vi "bigEncoder3.vi"(4 "Positive Direction":bool, 5 "ForceReset":bool, 7 "Allow C Reset?":bool=TRUE, 8 "Reset Array":bool[](array[boolean])=[FALSE, FALSE, FALSE], 11 "Encoder Array":bool[](array[boolean])=[FALSE, FALSE, FALSE]) -> (0 "Reseting":bool, 1 "JumpBy2Bit":bool, 2 "JumpBy2Error":i16, 3 "Position":i32)   [LabVIEW 2016, in "KevLib01.lvlib"]
uses:
  KevLib01.lvlib
panel:
  # "The Main Difference is I added Allowable C Reset"
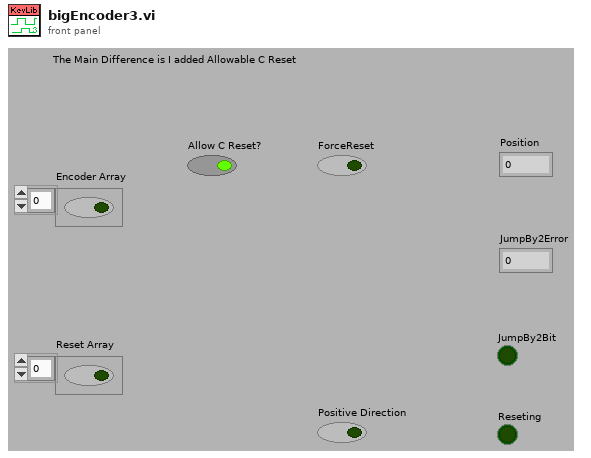
[diagram p1: front panel]
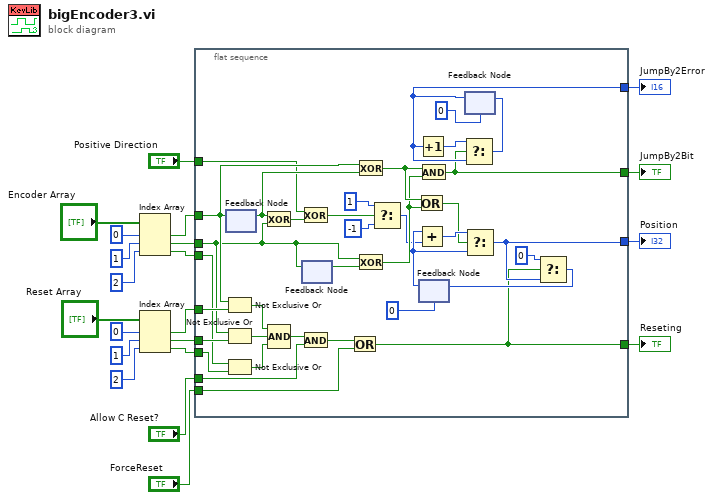
[diagram p0: block diagram]
diagram:
  n1 = Index Array(array="Encoder Array", index #1=0 ("index"), index #2=1 ("index"), index #3=2 ("index")) -> (element #1=w9:bool, element #2=w8:bool, element #3=w7:bool)
  n2 = Index Array(array="Reset Array", index #1=0 ("index"), index #2=1 ("index"), index #3=2 ("index")) -> (element #1=w6:bool, element #2=w5:bool, element #3=w4:bool)
  n3 = flat-sequence {
    tunnel: w9 -> [w37]
    tunnel: w8 -> [w35]
    tunnel: [w42] -> w21
    tunnel: [w45] -> w20
    tunnel: "ForceReset" -> [w39]
    tunnel: w6 -> [w38]
    tunnel: w5 -> [w36]
    tunnel: w4 -> [w34]
    tunnel: w7 -> [w33]
    tunnel: "Positive Direction" -> [w27]
    tunnel: [w26] -> w3
    tunnel: [w25] -> w2
    tunnel: "Allow C Reset?" -> [w23]
    frame #0 {
      n4 = Not Exclusive Or(1:w38, 2:w37) -> (0:w32:bool)
      n5 = Not Exclusive Or(1:w36, 2:w35) -> (0:w31:bool)
      n6 = Not Exclusive Or(1:w34, 2:w33) -> (0:w30:bool)
      n7 = feedback-in #1(w37) -> ()
      n8 = feedback #1() -> (w56:bool)  [unwired: 1 out]
      n9 = Exclusive Or(1:w35, 2:w56) -> (0:w29:bool)
      n10 = Compound Arithmetic op=AND(w32, w31, w30) -> (w24:bool)
      n11 = Exclusive Or(1:w29, 2:w27) -> (0:w28:bool)
      n12 = And(x=w24, y=w23) -> (x .and. y?=w22:bool)
      n13 = feedback-in #2(w35) -> ()
      n14 = feedback #2() -> (w57:bool)  [unwired: 1 out]
      n15 = Or(x=w22, y=w39) -> (x .or. y?=w26:bool)
      n16 = Exclusive Or(1:w56, 2:w37) -> (0:w50:bool)
      n17 = Exclusive Or(1:w57, 2:w35) -> (0:w49:bool)
      n18 = Select(t=1, s=w28, f=-1) -> (s? t:f=w43:i32)
      n19 = Or(x=w50, y=w49) -> (x .or. y?=w44:bool)
      n20 = And(x=w50, y=w49) -> (x .and. y?=w25:bool)
      n21 = feedback #3(0) -> (w51:i32)
      n22 = Add(x=w51, y=w43) -> (x+y=w55:i32)
      n23 = feedback #4(i16 0) -> (w45:i16)
      n24 = Increment(x=w45) -> (x+1=w47:i16)
      n25 = Select(t=w47, s=w25, f=w45) -> (s? t:f=w46:i16)
      n26 = feedback-in #4(w46) -> ()
      n27 = Select(t=w55, s=w44, f=w51) -> (s? t:f=w42:i32)
      n28 = Select(t=0, s=w26, f=w42) -> (s? t:f=w40:i32)
      n29 = feedback-in #3(w40) -> ()
    }
  }
  "Position" <- w21
  "JumpBy2Error" <- w20
  "Reseting" <- w3
  "JumpBy2Bit" <- w2
